vi "Schedule.Selector.vi"(8 "error in (no error)":errorcluster, 9 "Settings In":string, 10 "Schedule":u16, 11 "ObjectSettings in":refnum<class "ObjectSettings.lvclass">) -> (0 "error out":errorcluster, 1 "Settings Out":string, 3 "ObjectSettings out":refnum<class "ObjectSettings.lvclass">)   [LabVIEW 2019, in "ObjectSettings.lvclass"]
uses:
  ObjectSettings.lvclass
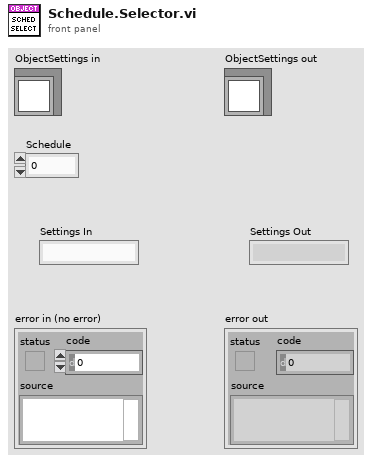
[diagram p1: front panel]
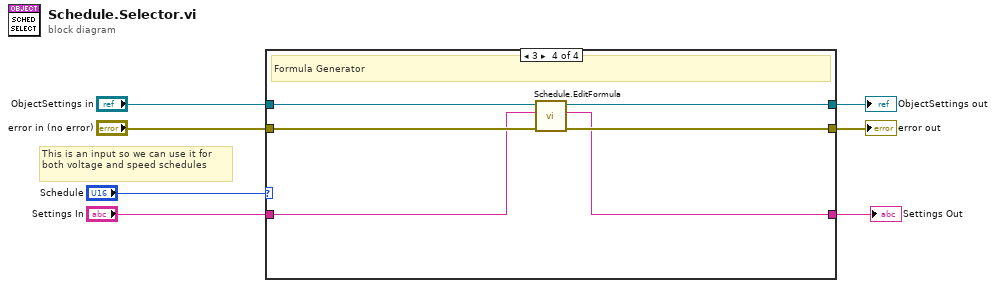
[diagram p0: block diagram]
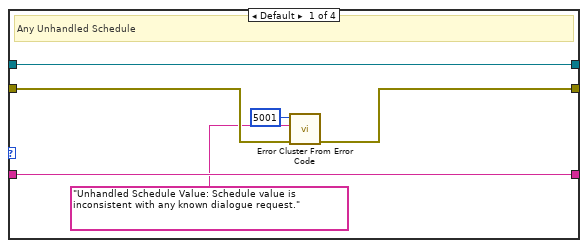
[diagram p2: hidden frame]
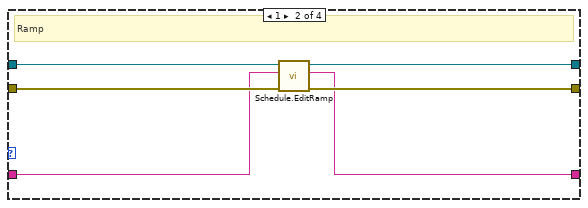
[diagram p3: hidden frame]
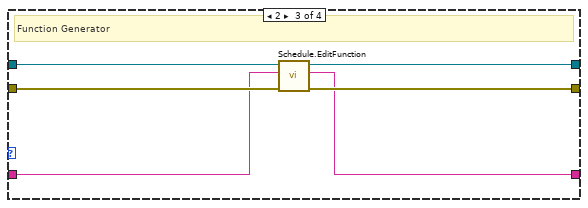
[diagram p4: hidden frame]
diagram:
  # "This is an input so we can use it for both voltage and speed schedules"
  n1 = case shown="3" "Schedule" {
    tunnel: "ObjectSettings in" -> [w13 w19 w24 w30]
    tunnel: [w13 w18 w25 w31] -> w5
    tunnel: "error in (no error)" -> [w10 w17 w22 w29]
    tunnel: [w11 w16 w23 w28] -> w3
    tunnel: "Settings In" -> [w12 w15 w20 w26]
    tunnel: [w12 w14 w21 w27] -> w1
    frame Default {
      # "Any Unhandled Schedule"
      n2 = call <vilib>:"Error Cluster From Error Code.vi"("error in (no error)"=w10, "error message (\"\")"="Unhandled Schedule Value: Schedule value is inconsistent with any known dialogue request." ("error message (\"\")"), "error code (0)"=5001) -> ("error out"=w11:errorcluster)  [unwired: 6 in]
    }
    frame 1 {
      # "Ramp"
      n3 = call-dynamic "Schedule.EditRamp.vi"("error in (no error)"=w17, "Settings"=w15, "ObjectSettings in"=w19) -> ("error out"=w16:errorcluster, "Settings Out"=w14:string, "ObjectSettings out"=w18:refnum<class "ObjectSettings.lvclass">)  [unwired: 6 in]
    }
    frame 2 {
      # "Function Generator"
      n4 = call-dynamic "Schedule.EditFunction.vi"("error in (no error)"=w22, "Settings"=w20, "ObjectSettings in"=w24) -> ("error out"=w23:errorcluster, "Settings Out"=w21:string, "ObjectSettings out"=w25:refnum<class "ObjectSettings.lvclass">)  [unwired: 6 in]
    }
    frame 3 {
      # "Formula Generator"
      n5 = call-dynamic "Schedule.EditFormula.vi"("error in (no error)"=w29, "Settings"=w26, "ObjectSettings in"=w30) -> ("error out"=w28:errorcluster, "Settings Out"=w27:string, "ObjectSettings out"=w31:refnum<class "ObjectSettings.lvclass">)  [unwired: 6 in]
    }
  }
  "error out" <- w3
  "ObjectSettings out" <- w5
  "Settings Out" <- w1
